vi "FTW-Scripter-Core_LoadScript.vi"(0 "FTW-Scripter-Core In":refnum<class "FTW-Scripter-Core.lvclass">, 5 "Script":string, 11 "error in":errorcluster) -> (4 "FTW-Scripter-Core Out":refnum<class "FTW-Scripter-Core.lvclass">, 15 "error out":errorcluster)   [LabVIEW 2015, in "FTW-Scripter-Core.lvclass"]
uses:
  FTW-Scripter-Core.lvclass
  FTW-Scripter-Core.lvclass/FTW-Scripter-Core.ctl
  source/container/FTW-Container.lvclass
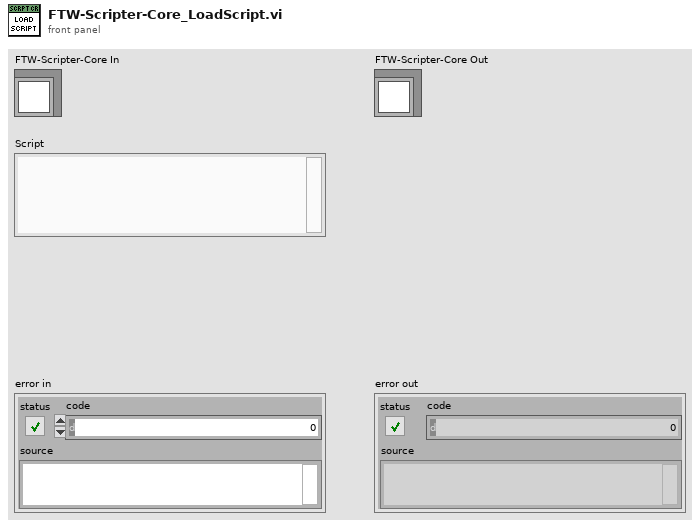
[diagram p1: front panel]
types:
  T1 = enum8{"Unloaded", "Loaded", "Executing", "Paused"}
  T2 = cluster{"Name":string, "Type":string, "Path":string, "Config":string}[]
  T3 = cluster{"Name":string, "Type":string, "Path":string, "Config":string}
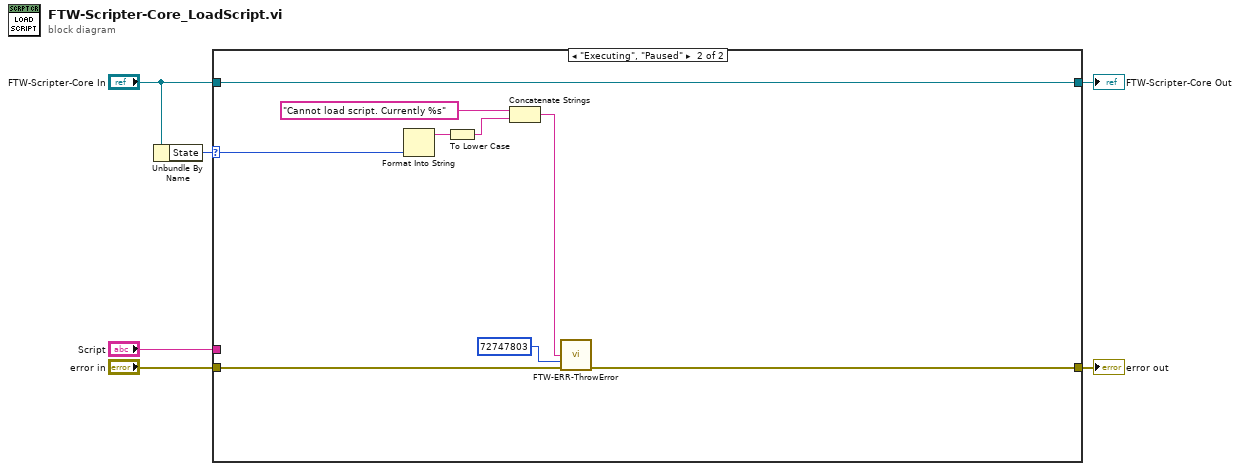
[diagram p0: block diagram]
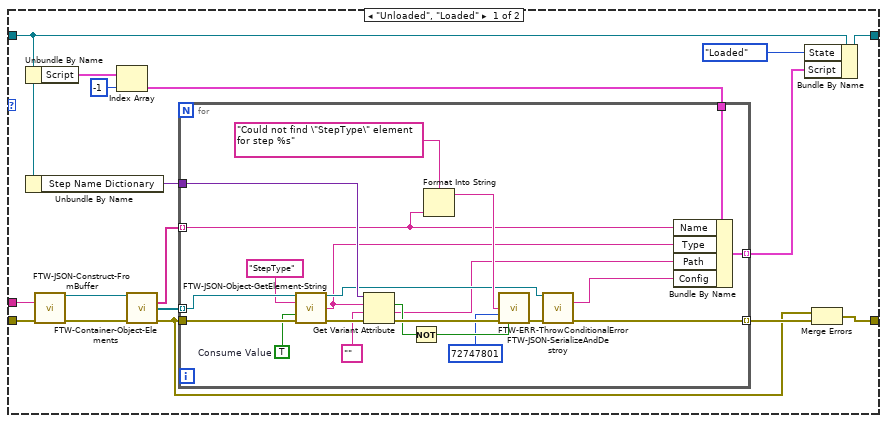
[diagram p2: hidden frame]
diagram:
  n1 = Unbundle By Name("FTW-Scripter-Core In") -> ("State"=w4:T1)
  n2 = case shown="\"Executing\", \"Paused\"" w4 {
    selector: w4 -> [_ w50]
    tunnel: [w22 w54] -> w6
    tunnel: "FTW-Scripter-Core In" -> [w10 w54]
    tunnel: [w12 w52] -> w3
    tunnel: "error in" -> [w23 w53]
    tunnel: "Script" -> [w19 _]
    frame "Unloaded", "Loaded" {
      n3 = Unbundle By Name(w10) -> ("Script"=w9:T2)
      n4 = Unbundle By Name(w10) -> ("Step Name Dictionary"=w16:variant)
      n5 = call "FTW-JSON-Construct-FromBuffer.vi"("JSON String (UTF-8)"=w19, "error in"=w23) -> ("JSON"=w18:refnum<class "FTW-Container.lvclass">, "error out"=w20:errorcluster)  [unwired: 12 in]
      n6 = Index Array(array=w9, index=-1) -> (element=w7:T3)
      n7 = call "FTW-Container-Object-Elements.vi"("FTW-Container In"=w18, "error in"=w20) -> ("Names"=w21:string[], "Object Elements"=w17:refnum<class "FTW-Container.lvclass">[], "error out"=w11:errorcluster)  [unwired: 10 in, 1 out]
      n8 = for {
        tunnel: w21 -> [w29] mode=indexing
        tunnel: w11 -> [w44]
        tunnel: w17 -> [w45] mode=indexing
        tunnel: w16 -> [w39]
        tunnel: [w31] -> w13 mode=indexing
        tunnel: [w28] -> w15 mode=indexing
        tunnel: w7 -> [w24]
        w42 = TRUE  # Consume Value
        n9 = call "FTW-JSON-Object-GetElement-String.vi"("JSON"=w45, "Key"="StepType", "Consume Value"=w42, "error in"=w44) -> ("JSON out"=w30:refnum<class "FTW-Container.lvclass">, "Value"=w26:string, "error out"=w41:errorcluster)  [unwired: 7 in, 2 out]
        n10 = Get Variant Attribute(Variant=w39, name=w26, default value (empty Variant)="" ("empty string"), error in=w41) -> (found=w36:bool, value=w25:string, error out=w38:errorcluster)  [unwired: 1 out]
        n11 = Not(x=w36) -> (.not. x?=w35:bool)
        n12 = Format Into String(format string="Could not find \"StepType\" element for step %s" ("Error Message"), w29) -> (resulting string=w33:string)  [unwired: 2 in, 1 out]
        n13 = call "FTW-ERR-ThrowConditionalError.vi"("Error Message"=w33, "Error Code"=72747801, "error in"=w38, "Throw Error?"=w35) -> ("error out"=w37:errorcluster)  [unwired: 11 in]
        n14 = call "FTW-JSON-SerializeAndDestroy.vi"("JSON"=w30, "error in"=w37) -> ("JSON String (UTF-8)"=w27:string, "error out"=w31:errorcluster)  [unwired: 12 in]
        n15 = Bundle By Name(cluster=w24, "Name"=w29, "Type"=w26, "Path"=w25, "Config"=w27) -> (w28:T3)
      }
      n16 = Bundle By Name(cluster=w10, "State"=T1."Loaded", "Script"=w15) -> (w22:refnum<class "FTW-Scripter-Core.lvclass">)
      n17 = Merge Errors(w11, w13) -> (w12:errorcluster)
    }
    frame "Executing", "Paused" {
      n18 = Format Into String(w50) -> (resulting string=w49:string)  [unwired: 3 in, 1 out]
      n19 = To Lower Case(string=w49) -> (all lower case string=w47:string)
      n20 = Concatenate Strings("Cannot load script. Currently %s" ("Error Message"), w47) -> (w48:string)
      n21 = call "FTW-ERR-ThrowError.vi"("Error Message"=w48, "Error Code"=72747803, "error in"=w53) -> ("error out"=w52:errorcluster)  [unwired: 12 in]
    }
  }
  "FTW-Scripter-Core Out" <- w6
  "error out" <- w3
